vi "BSA_Monitor.vi"() -> ()   [LabVIEW 2010]
uses:
  Globals/LDA_meas_global_1.vi
panel:
  out "error out":errorcluster
  in  "BSASysMon.IBSASysMon":refnum<k7>(container)
  in  "stop":bool
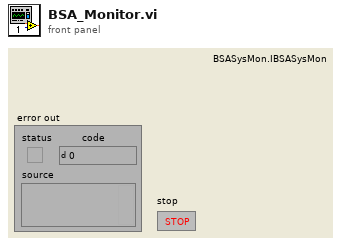
[diagram p1: front panel]
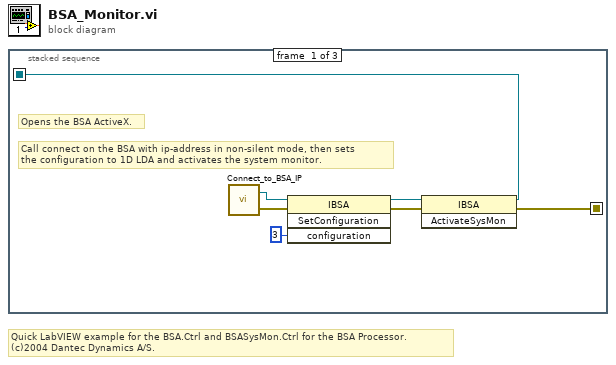
[diagram p0: block diagram]
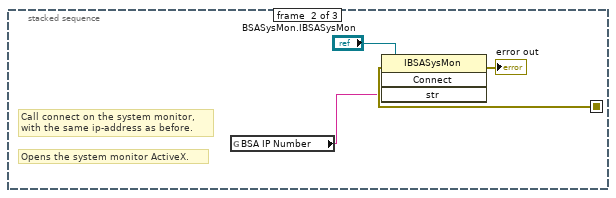
[diagram p2: hidden frame]
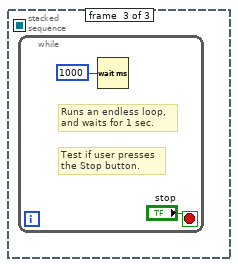
[diagram p3: hidden frame]
diagram:
  # "Quick LabVIEW example for the BSA.Ctrl and BSASysMon.Ctrl for the BSA Processor.\n(c)2004 Dantec Dynamics A/S."
  n1 = stacked-sequence {
    seq-local: [w4 _ _] -> [_ w11 _]
    seq-local: [w1 _ _] -> [_ _ _]
    frame #0 {
      # "Call connect on the BSA with ip-address in non-silent mode, then sets\nthe configuration to 1D LDA and activates the system monitor."
      # "Opens the BSA ActiveX."
      n2 = call "Connect_to_BSA_IP.vi"() -> ("error out"=w2:errorcluster, "BSA"=w3:refnum<k7>)  [unwired: 2 out]
      n3 = invoke class="IBSA" method="SetConfiguration"(reference=w3, error in=w2, "configuration"=3 ("config")) -> (reference out=w7:refnum<k7>, error out=w5:errorcluster)  [unwired: 1 in, 2 out]
      n4 = invoke class="IBSA" method="ActivateSysMon"(reference=w7, error in=w5) -> (reference out=w1:refnum<k7>, error out=w4:errorcluster)  [unwired: 1 in, 1 out]
    }
    frame #1 {
      # "Call connect on the system monitor,\nwith the same ip-address as before."
      # "Opens the system monitor ActiveX."
      n5 = global read "LDA_meas_global_1.vi" "BSA IP Number"() -> (w9:string)
      n6 = invoke class="IBSASysMon" method="Connect"(reference="BSASysMon.IBSASysMon", error in=w11, "str"=w9) -> (error out=→"error out":errorcluster)  [unwired: 1 in, 3 out]
    }
    frame #2 {
      n7 = while {
        stop <- "stop" stop-if-true
        # "Test if user presses\nthe Stop button."
        # "Runs an endless loop,\nand waits for 1 sec."
        n8 = Wait (ms)(milliseconds to wait=u32 1000) -> ()  [unwired: 1 out]
      }
    }
  }
